vi "maszyna stanowa 1.vi"() -> ()   [LabVIEW 2014]
uses:
  sklep.ctl
  event.ctl
panel:
  out "liczba klientów":i32
  out "zarobek":i32
  out "średni czas w kolejce":dbl
  out "Sklep 2":T1
  in  "Sklep":T1
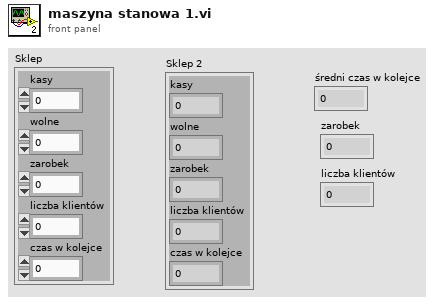
[diagram p1: front panel]
types:
  T1 = typedef "sklep.ctl" = cluster{"kasy":i32, "wolne":i32, "zarobek":i32, "liczba klientów":i32, "czas w kolejce":i32}
  T2 = typedef "event.ctl" = cluster{"czas":u32, "event":enum16{"przyjście klienata", "zwolnienie kasy", "oczekiwanie na klienta", "nowy event"}}
  T3 = enum16{"przyjście klienata", "zwolnienie kasy", "oczekiwanie na klienta", "nowy event"}
  T4 = cluster{dbl, "event":enum16{"przyjście klienata", "zwolnienie kasy", "oczekiwanie na klienta", "nowy event"}}
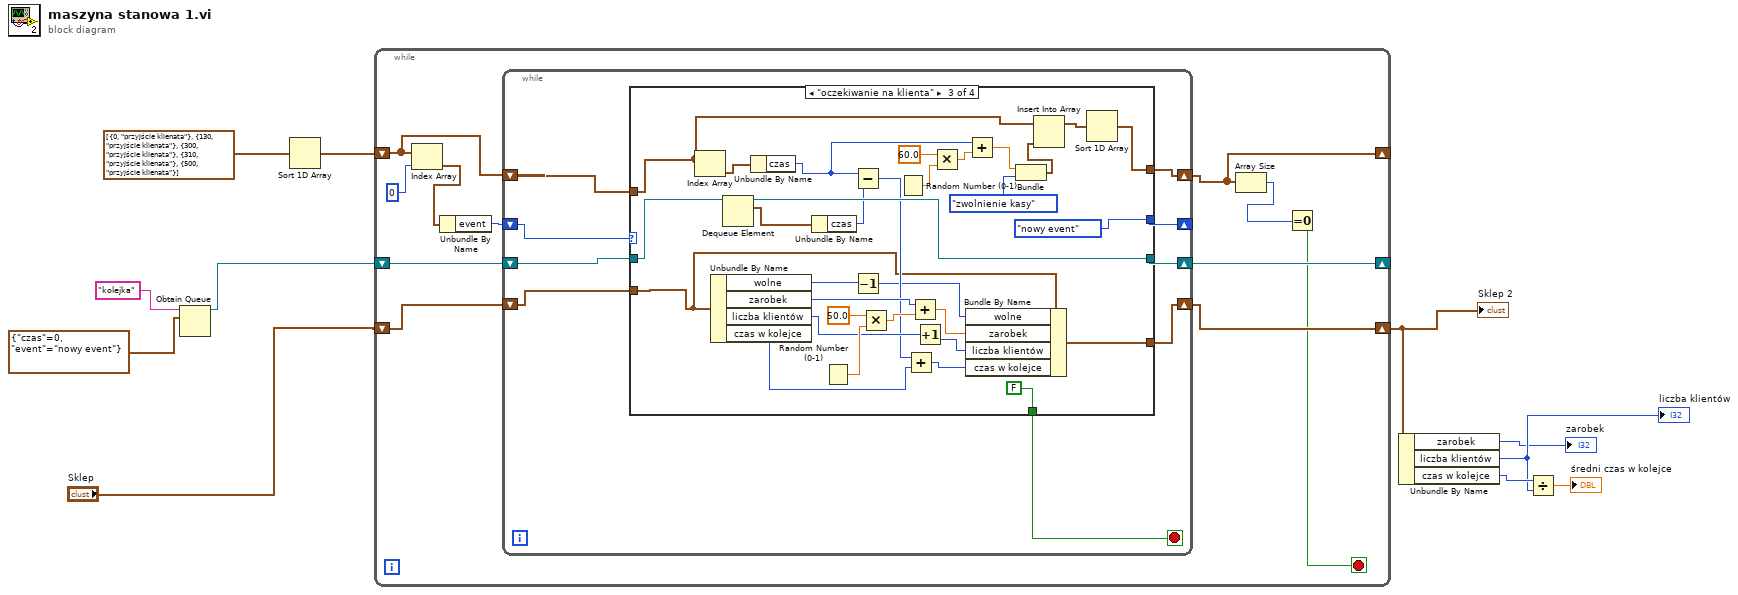
[diagram p0: block diagram]
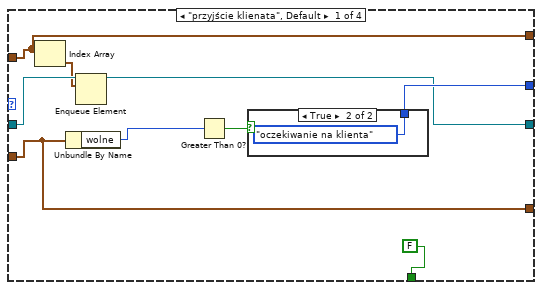
[diagram p2: hidden frame]
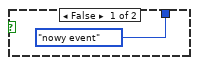
[diagram p3: hidden frame]
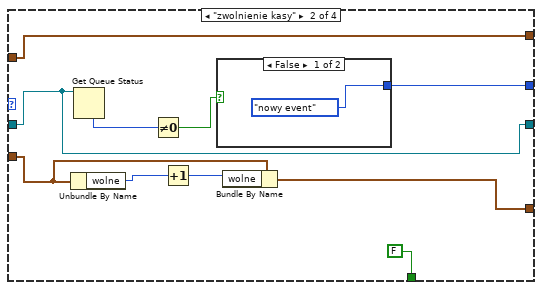
[diagram p4: hidden frame]
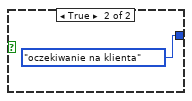
[diagram p5: hidden frame]
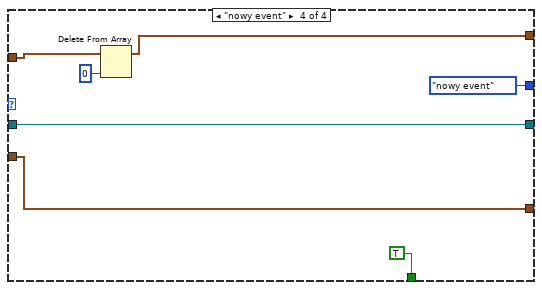
[diagram p6: hidden frame]
diagram:
  n1 = Obtain Queue(name (unnamed)="kolejka", element data type=T2 {"czas"=0, "event"=enum."nowy event"} ("Cluster")) -> (queue out=w7:refnum<queue>)  [unwired: 3 in, 2 out]
  n2 = Sort 1D Array(array=T2[] [{"czas"=0, "event"=enum."przyjście klienata"}, {"czas"=130, "event"=enum."przyjście klienata"}, {"czas"=300, "event"=enum."przyjście klienata"}, {"czas"=310, "event"=enum."przyjście klienata"}, {"czas"=500, "event"=enum."przyjście klienata"}]) -> (sorted array=w10:T2[])
  n3 = while {
    shift-right: [w15] -> w5
    shift-left: "Sklep" -> [w19]
    shift-right: [w16] -> _
    shift-left: w7 -> [w20]
    shift-right: [w12] -> _
    shift-left: w10 -> [w21]
    stop <- w13 stop-if-true
    n4 = Index Array(array=w21, index=0) -> (element=w18:T2)
    n5 = Unbundle By Name(w18) -> ("event"=w17:T3)
    n6 = while {
      shift-right: [w27] -> _
      shift-left: w17 -> [w28]
      shift-right: [w25] -> w15
      shift-left: w19 -> [w29]
      shift-right: [w26] -> w16
      shift-left: w20 -> [w30]
      shift-right: [w24] -> w12
      shift-left: w21 -> [w31]
      stop <- w23 stop-if-true
      n7 = case shown="\"oczekiwanie na klienta\"" w28 {
        tunnel: w31 -> [w34 w45 w65 w92]
        tunnel: w30 -> [w40 w43 w79 w88]
        tunnel: w29 -> [w33 w51 w72 w87]
        tunnel: [w36 w46 T3."nowy event" ("event") T3."nowy event" ("event")] -> w27
        tunnel: [w35 w43 w78 w88] -> w26
        tunnel: [w33 w49 w67 w87] -> w25
        tunnel: [w34 w45 w56 w90] -> w24
        tunnel: [FALSE FALSE FALSE TRUE] -> w23
        frame "przyjście klienata", Default {
          n8 = Index Array(array=w34) -> (element=w39:T2)  [unwired: 1 in]
          n9 = Unbundle By Name(w33) -> ("wolne"=w38:i32)
          n10 = Enqueue Element(queue=w40, element=w39) -> (queue out=w35:refnum<queue>)  [unwired: 2 in, 2 out]
          n11 = Greater Than 0?(x=w38) -> (x > 0?=w37:bool)
          n12 = case shown="True" w37 {
            tunnel: [T3."nowy event" ("event") T3."oczekiwanie na klienta" ("event")] -> w36
            frame False {
            }
            frame True {
            }
          }
        }
        frame "zwolnienie kasy" {
          n13 = Unbundle By Name(w51) -> ("wolne"=w52:i32)
          n14 = Get Queue Status(queue=w43) -> (# elements in queue=w48:i32)  [unwired: 2 in, 7 out]
          n15 = Not Equal To 0?(x=w48) -> (x != 0?=w47:bool)
          n16 = Increment(x=w52) -> (x+1=w50:i32)
          n17 = case shown="False" w47 {
            tunnel: [T3."nowy event" ("event") T3."oczekiwanie na klienta" ("event")] -> w46
            frame False {
            }
            frame True {
            }
          }
          n18 = Bundle By Name(cluster=w51, "wolne"=w50) -> (w49:T1)
        }
        frame "oczekiwanie na klienta" {
          n19 = Index Array(array=w65) -> (element=w76:T2)  [unwired: 1 in]
          n20 = Unbundle By Name(w72) -> ("wolne"=w85:i32, "zarobek"=w83:i32, "liczba klientów"=w80:i32, "czas w kolejce"=w74:i32)
          n21 = Dequeue Element(queue=w79) -> (queue out=w78:refnum<queue>, element=w77:T2)  [unwired: 2 in, 2 out]
          n22 = Unbundle By Name(w76) -> ("czas"=w64:u32)
          n23 = Unbundle By Name(w77) -> ("czas"=w75:u32)
          n24 = Random Number (0-1)() -> (number: 0 to 1=w82:dbl)
          n25 = Subtract(x=w64, y=w75) -> (x-y=w73:u32)
          n26 = Decrement(x=w85) -> (x-1=w71:i32)
          n27 = Multiply(x=50.0, y=w82) -> (x*y=w84:dbl)
          n28 = Random Number (0-1)() -> (number: 0 to 1=w61:dbl)
          n29 = Add(x=w73, y=w74) -> (x+y=w68:u32)
          n30 = Add(x=w83, y=w84) -> (x+y=w70:dbl)
          n31 = Increment(x=w80) -> (x+1=w69:i32)
          n32 = Multiply(x=60.0, y=w61) -> (x*y=w63:dbl)
          n33 = Bundle By Name(cluster=w72, "wolne"=w71, "zarobek"=w70, "liczba klientów"=w69, "czas w kolejce"=w68) -> (w67:T1)
          n34 = Add(x=w64, y=w63) -> (x+y=w60:dbl)
          n35 = Bundle(w60, "event"=T3."zwolnienie kasy") -> (w58:T4)  [unwired: 1 in]
          n36 = Insert Into Array(array=w65, new element=w58) -> (w57:T2[])  [unwired: 1 in]
          n37 = Sort 1D Array(array=w57) -> (sorted array=w56:T2[])
        }
        frame "nowy event" {
          n38 = Delete From Array(array=w92, index=0) -> (array with subset deleted=w90:T2[])  [unwired: 1 in, 1 out]
        }
      }
    }
    n39 = Array Size(array=w12) -> (size(s)=w14:i32)
    n40 = Equal To 0?(x=w14) -> (x = 0?=w13:bool)
  }
  "Sklep 2" <- w5
  n41 = Unbundle By Name(w5) -> ("zarobek"=→"zarobek":i32, "liczba klientów"=w3:i32, "czas w kolejce"=w4:i32)
  "liczba klientów" <- w3
  n42 = Divide(x=w4, y=w3) -> (x/y=→"średni czas w kolejce":dbl)
